vi "Problem1.9-RandomNumbers.vi"() -> ()   [LabVIEW 2019]
panel:
  out "Original Random Number Array":dbl[][](array[numeric])
  out "Uniform Deviates Array":dbl[][](array[numeric])
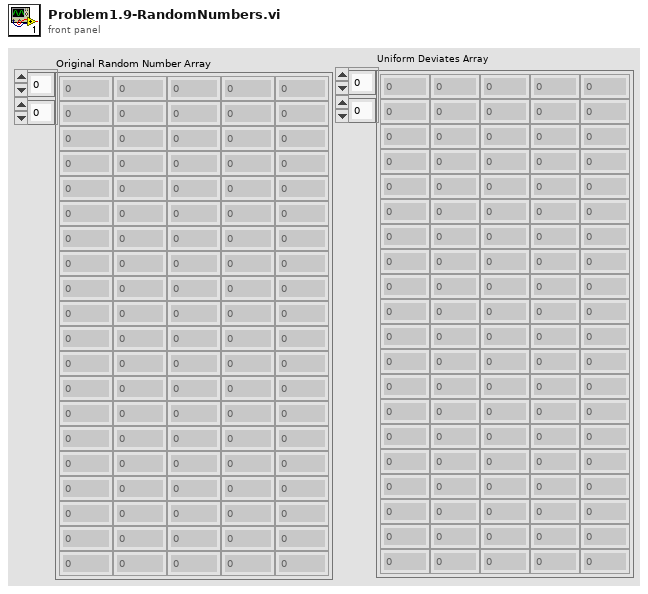
[diagram p1: front panel]
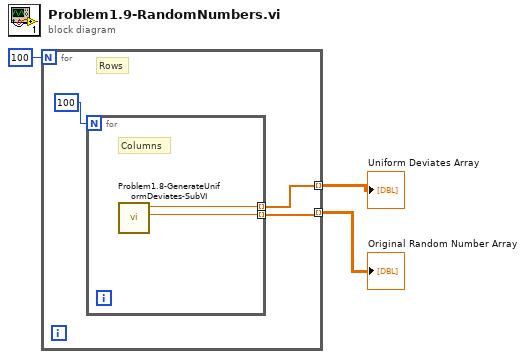
[diagram p0: block diagram]
diagram:
  n1 = for {
    N: 100 -> [_]
    tunnel: [w5] -> w2 mode=indexing
    tunnel: [w4] -> w1 mode=indexing
    # "Rows"
    n2 = for {
      N: 100 -> [_]
      tunnel: [w8] -> w5 mode=indexing
      tunnel: [w7] -> w4 mode=indexing
      # "Columns"
      n3 = call "Problem1.8-GenerateUniformDeviates-SubVI.vi"() -> ("number: 0 to 1"=w7:dbl, "Numeric"=w8:dbl)  [unwired: 10 in]
    }
  }
  "Uniform Deviates Array" <- w2
  "Original Random Number Array" <- w1
